vi "Configure Power Measurement Result Mode.vi"(8 "error in (no error)":errorcluster, 9 "Mode (Power)":i32(ring) items=["Power", "Statistic"], 10 "Instance (1)":i32=1, 11 "VISA resource name":refnum<visa-resource-name>) -> (0 "error out":errorcluster, 3 "VISA resource name out":refnum<visa-resource-name>)   [LabVIEW 2020, in "Rohde&Schwarz CMXP GPRF.lvlib"]
doc: "This VI sets the result mode for the single step power measurement.\n\nAttribute:\nRSCMXPGPRF_ATTR_POWER_MEASUREMENT_RESULT_MODE\n\nRemote-control command:\nCONFigure:GPRF:MEAS<i>:POWer:MODE"
uses:
  <instrlib>/Rohde&Schwarz CMXP GPRF/Rohde&Schwarz CMXP GPRF.lvlib
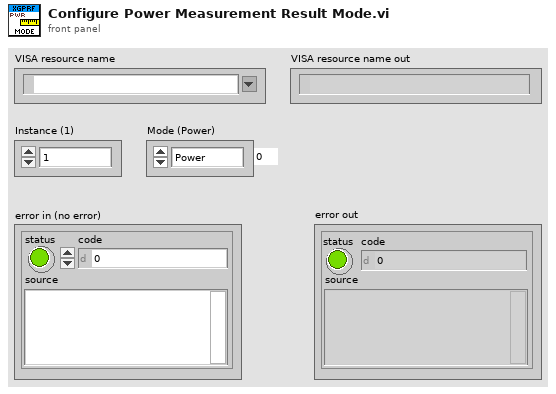
[diagram p1: front panel]
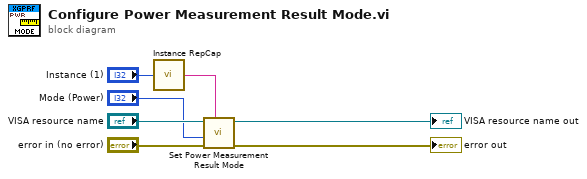
[diagram p0: block diagram]
diagram:
  n1 = call <instrlib>:"Instance RepCap.vi"("Instance in"="Instance (1)") -> ("Instance out"=w7:string)
  n2 = call "Set Power Measurement Result Mode"("Repeated Capabilities"=w7, "error in (no error)"="error in (no error)", "Power Measurement Result Mode (0 - Power)"="Mode (Power)", "instrument handle"="VISA resource name") -> ("error out"=→"error out":errorcluster, "instrument handle out"=→"VISA resource name out":refnum<visa-resource-name>)  [unwired: 6 in]
